vi "Clear_Devices.vi"(8 "error in (no error)":errorcluster) -> (0 "error out":errorcluster)   [LabVIEW 2012]
doc: "Closes handles and clears records of unplugged devices."
uses:
  Windows/System32/AIOUSB.dll
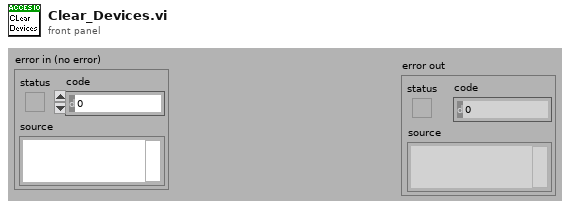
[diagram p1: front panel]
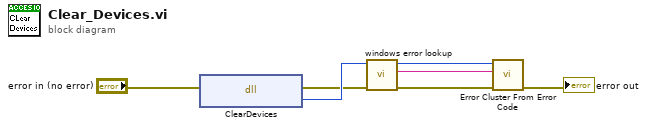
[diagram p0: block diagram]
diagram:
  n1 = dll-call lib="C:/Windows/System32/AIOUSB.dll" fn="ClearDevices"(error in="error in (no error)") -> (error out=w2:errorcluster, "return type"=w3:u32)  [unwired: 2 in, 1 out]
  n2 = call "windows error lookup.vi"("error in (no error)"=w2, "Error Code"=w3) -> ("error out"=w1:errorcluster, "error message (\"\")"=w4:string)  [unwired: 8 in]
  n3 = call <vilib>:"Error Cluster From Error Code.vi"("error in (no error)"=w1, "error message (\"\")"=w4, "error code (0)"=w3) -> ("error out"=→"error out":errorcluster)  [unwired: 6 in]
